vi "BundelbyName.vi"() -> ()   [LabVIEW 2021]
panel:
  out "IndEmp":T1
  in  "Cluster":T1
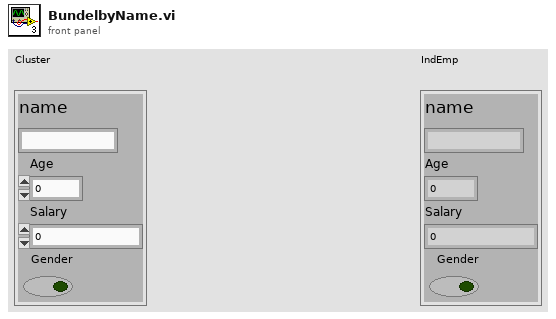
[diagram p1: front panel]
types:
  T1 = cluster{"name":string, "Age":u8, "Salary":u32, "Gender":bool}
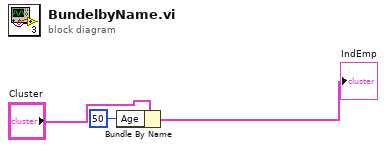
[diagram p0: block diagram]
diagram:
  n1 = Bundle By Name(cluster="Cluster", "Age"=u8 50) -> (→"IndEmp":T1)
